vi "SaveFile.vi"(8 "error in (no error)":errorcluster, 9 "Data":string, 10 "Filename":string, 11 "TCP_Server_Connection_Handler in":refnum<class "TCP_Server_Connection_Handler.lvclass">) -> (0 "error out":errorcluster, 3 "TCP_Server_Connection_Handler out":refnum<class "TCP_Server_Connection_Handler.lvclass">)   [LabVIEW 2023, in "TCP_Server_Connection_Handler.lvlib" / "TCP_Server_Connection_Handler.lvclass"]
uses:
  TCP_Server_Connection_Handler.lvclass
  <vilib>/ActorFramework/Actor/Actor.lvclass/Actor.ctl
  <vilib>/ActorFramework/Message Enqueuer/Message Enqueuer.lvclass/Message Enqueuer.ctl
  TCP_Server_Connection_Handler.lvclass/TCP_Server_Connection_Handler.ctl
  <vilib>/Utility/error.llb/DialogType.ctl
  TCP_Server_Connection_Handler Messages/SendString Msg/SendString Msg.lvclass/SendString Msg.ctl
  <vilib>/ActorFramework/Message Enqueuer/Init from Existing Queue.vi
  <vilib>/ActorFramework/Message Enqueuer/Enqueue.vi
  TCP_Server_Connection_Handler Messages/SendString Msg/SendString Msg.lvclass
  <vilib>/ActorFramework/Message Priority Queue/Priority Enqueue.vi
  <vilib>/ActorFramework/Message Enqueuer/Message Enqueuer.lvclass
  <vilib>/ActorFramework/Actor/Actor.lvclass
  TypeDefinitions/messageType.ctl
  TCP_Server_Connection_Handler.lvlib
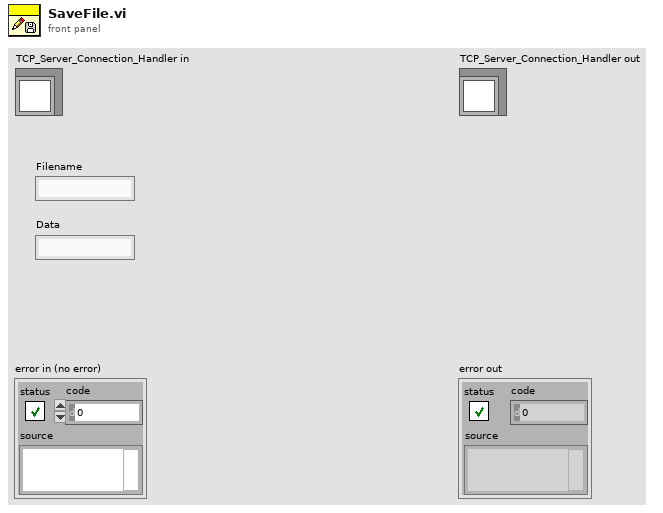
[diagram p1: front panel]
types:
  T1 = typedef "TCP_Server_Connection_Handler.lvlib/messageType.ctl" = enum16{"message", "file", "get", "ShutDown"}
  T2 = enum16{"open", "replace", "create", "open or create", "replace or create", "replace or create with confirmation"}
  T3 = typedef "DialogType.ctl" = u16
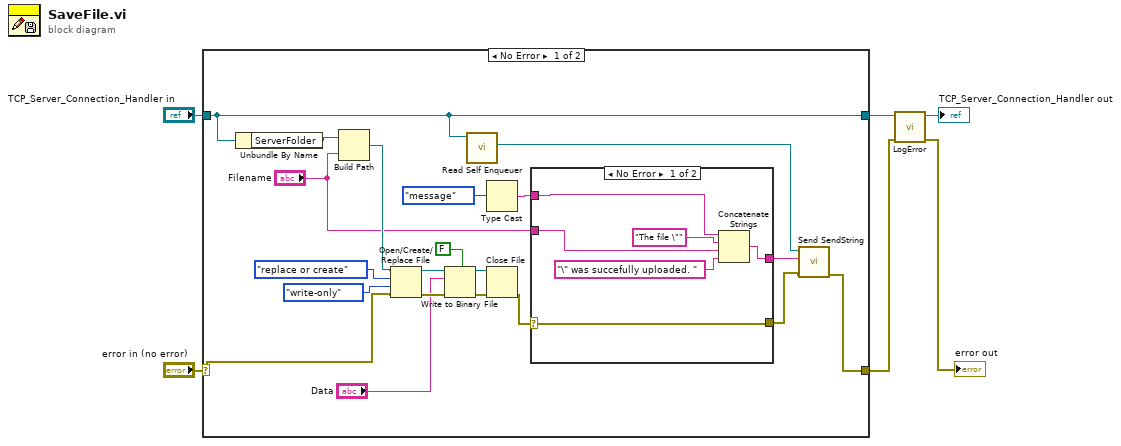
[diagram p0: block diagram]
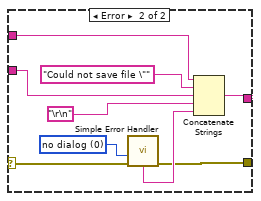
[diagram p2: hidden frame]
diagram:
  n1 = case shown="No Error" "error in (no error)" {
    selector: "error in (no error)" -> [w17 w43]
    tunnel: [w11 w43] -> w2
    tunnel: [w10 w42] -> w4
    tunnel: "TCP_Server_Connection_Handler in" -> [w10 w42]
    frame No Error {
      n2 = Unbundle By Name(w10) -> ("ServerFolder"=w26:path)
      n3 = Build Path(base path=w26, name or relative path="Filename") -> (appended path=w25:path)
      n4 = Open/Create/Replace File(file path (use dialog)=w25, error in=w17, operation (0:open)=T2."replace or create", access (0:read/write)=enum16{"read/write", "read-only", "write-only"}."write-only") -> (refnum out=w22:refnum<file>, error out=w21:errorcluster)  [unwired: 2 in, 1 out]
      n5 = Write to Binary File(file (use dialog)=w22, data="Data", error in=w21, 5:FALSE ("prepend array or string size? (T)")) -> (refnum out=w19:refnum<file>, error out=w20:errorcluster)  [unwired: 2 in, 1 out]
      n6 = call <vilib>:"Read Self Enqueuer.vi"("Actor"=w10) -> ("Self Enqueuer"=w12:refnum<class "Message Enqueuer.lvclass">)  [unwired: 10 in]
      n7 = Type Cast(x=messageType."message" ("MessageType")) -> (*(type *) &x=w7:string)  [unwired: 1 in]
      n8 = Close File(refnum=w19, error in=w20) -> (error out=w15:errorcluster)  [unwired: 1 out]
      n9 = case shown="No Error" w15 {
        selector: w15 -> [w28 w38]
        tunnel: "Filename" -> [w31 w40]
        tunnel: [w28 w34] -> w9
        tunnel: [w29 w35] -> w13
        tunnel: w7 -> [w27 w33]
        frame No Error {
          n10 = Concatenate Strings(w27, "The file \"", w31, "\" was succefully uploaded. " ("string")) -> (w29:string)
        }
        frame Error {
          w36 = T3 0 items=["no dialog", "OK message", "continue or stop message", "OK message + warnings", "continue/stop + warnings"] ("type of dialog (OK msg:1)")
          n11 = call <vilib>:"Simple Error Handler.vi"("type of dialog (OK msg:1)"=w36, "error in (no error)"=w38) -> ("error out"=w34:errorcluster, "message"=w37:string)  [unwired: 3 in, 3 out]
          n12 = Concatenate Strings(w33, "Could not save file \"", w40, "\r\n", w37) -> (w35:string)
        }
      }
      n13 = call "Send SendString.vi"("error in (no error)"=w9, "Message"=w13, "Message Enqueuer"=w12) -> ("error out"=w11:errorcluster)  [unwired: 7 in, 1 out]
    }
    frame Error {
    }
  }
  n14 = call "LogError.vi"("error in (no error)"=w2, "TCP_Server_Connection_Handler in"=w4) -> ("error out"=→"error out":errorcluster, "TCP_Server_Connection_Handler out"=→"TCP_Server_Connection_Handler out":refnum<class "TCP_Server_Connection_Handler.lvclass">)  [unwired: 8 in]
